vi "New.vi"(8 "error in (no error)":errorcluster, 11 "reference in":refnum<class "MES_Local.lvclass">) -> (0 "error out":errorcluster, 3 "reference out":refnum<class "MES_Local.lvclass">)   [LabVIEW 2022 SP3, in "MES_Local.lvlib" / "MES_Local.lvclass"]
uses:
  MES_Local.lvclass
  ObjectAttributes.ctl
  Components/Login_Base.lvlibp/Login_Base.lvclass
  Config.ctl
  Components/MES_Base.lvlibp/Controls/Spec.ctl
  MES_Local.lvclass/MES_Local.ctl
  Components/MES_Base.lvlibp/MES_Base.lvclass
panel:
  in  "Data":T1
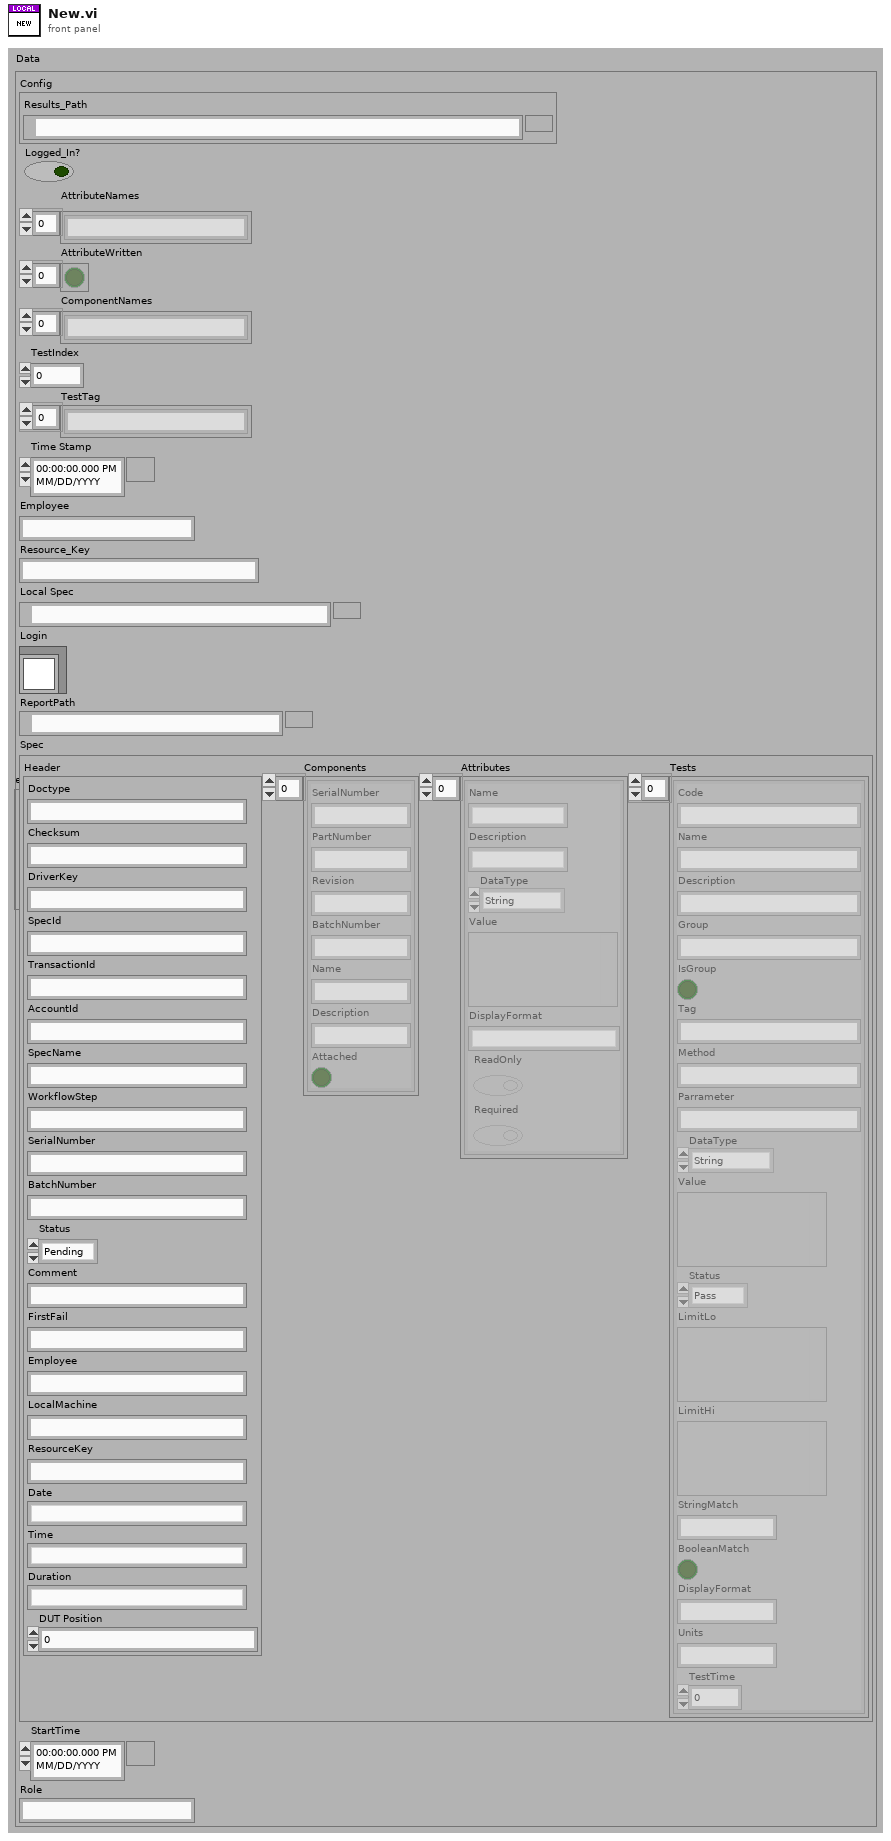
[diagram p1: front panel]
types:
  T1 = typedef "MES_Local.lvlib/MES_Local.lvclass/ObjectAttributes.ctl" = cluster{"Config":T2, "Logged_In?":bool, "AttributeNames":string[], "AttributeWritten":bool[], "ComponentNames":string[], "TestIndex":i32, "TestTag":string[], "Time Stamp":timestamp, "Employee":string, "Resource_Key":string, "Local Spec":path, "Login":refnum<class "Login_Base.lvclass">, "ReportPath":path, "Spec":T3, "StartTime":timestamp, "Role":string}
  T2 = typedef "MES_Local.lvlib/MES_Local.lvclass/Config.ctl" = cluster{"Results_Path":path}
  T3 = typedef "MES_Base.lvlibp/MES_Base.lvclass/Spec.ctl" = cluster{"Header":cluster{"Doctype":string, "Checksum":string, "DriverKey":string, "SpecId":string, "TransactionId":string, "AccountId":string, "SpecName":string, "WorkflowStep":string, "SerialNumber":string, "BatchNumber":string, "Status":enum16{"Pending", "Pass", "Fail"}, "Comment":string, "FirstFail":string, "Employee":string, "LocalMachine":string, "ResourceKey":string, "Date":string, "Time":string, "Duration":string, "DUT Position":i32}, "Components":cluster{"SerialNumber":string, "PartNumber":string, "Revision":string, "BatchNumber":string, "Name":string, "Description":string, "Attached":bool}[], "Attributes":cluster{"Name":string, "Description":string, "DataType":enum16{"NA", "String", "Boolean", "Int", "Dbl"}, "Value":variant, "DisplayFormat":string, "ReadOnly":bool, "Required":bool}[], "Tests":cluster{"Code":string, "Name":string, "Description":string, "Group":string, "IsGroup":bool, "Tag":string, "Method":string, "Parrameter":string, "DataType":enum16{"NA", "String", "Boolean", "Int", "Dbl"}, "Value":variant, "Status":enum16{"Pending", "Pass", "Fail"}, "LimitLo":variant, "LimitHi":variant, "StringMatch":string, "BooleanMatch":bool, "DisplayFormat":string, "Units":string, "TestTime":dbl}[]}
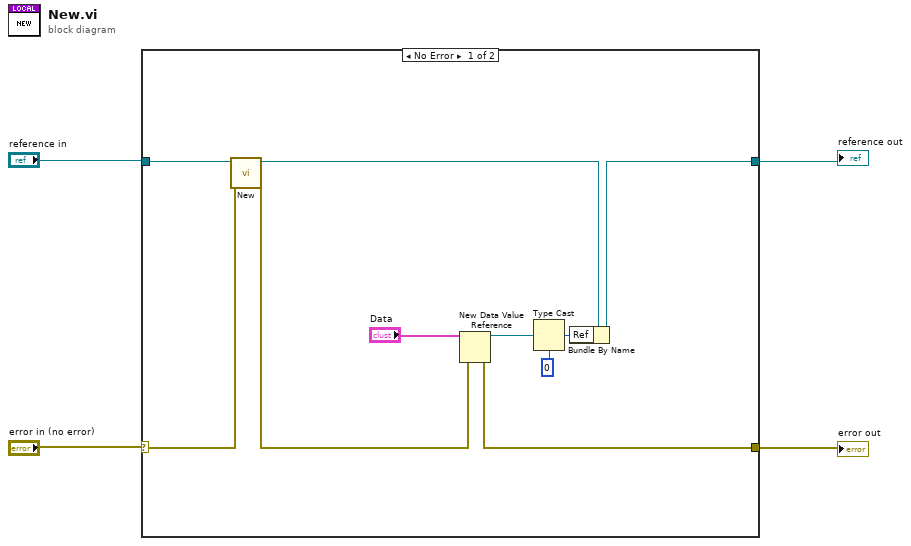
[diagram p0: block diagram]
diagram:
  n1 = case shown="No Error" "error in (no error)" {
    selector: "error in (no error)" -> [w8 w16]
    tunnel: [w6 w16] -> w2
    tunnel: "reference in" -> [w14 w15]
    tunnel: [w13 w15] -> w1
    frame No Error {
      n2 = call-parent "New.vi"("error in (no error)"=w8, "reference in"=w14) -> ("error out"=w7:errorcluster, "reference out"=w12:refnum<class "MES_Local.lvclass">)  [unwired: 8 in]
      n3 = New Data Value Reference(data value="Data", error in=w7) -> (data value reference=w10:refnum<data-value>, error out=w6:errorcluster)
      n4 = Type Cast(type=u32 0 ("DataRef"), x=w10) -> (*(type *) &x=w9:u32)
      n5 = Bundle By Name(cluster=w12, "Ref"=w9) -> (w13:refnum<class "MES_Local.lvclass">)
    }
    frame Error {
    }
  }
  "error out" <- w2
  "reference out" <- w1
